vi "Stop_queue.vi"(7 "Refs cluster In":T1) -> ()   [LabVIEW 2015]
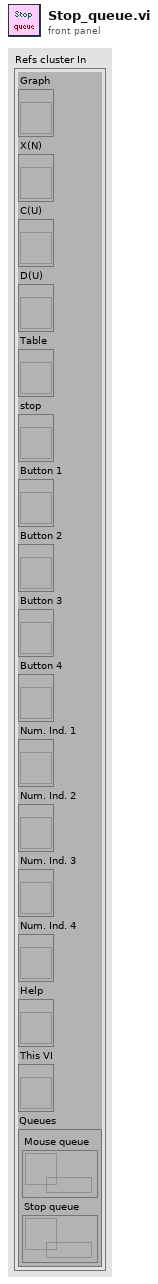
[diagram p1: front panel]
types:
  T1 = cluster{"Graph":refnum<vi>, "X(N)":refnum<vi>, "C(U)":refnum<vi>, "D(U)":refnum<vi>, "Table":refnum<vi>, "stop":refnum<vi>, "Button 1":refnum<vi>, "Button 2":refnum<vi>, "Button 3":refnum<vi>, "Button 4":refnum<vi>, "Num. Ind. 1":refnum<vi>, "Num. Ind. 2":refnum<vi>, "Num. Ind. 3":refnum<vi>, "Num. Ind. 4":refnum<vi>, "Help":refnum<vi>, "This VI":refnum<vi>, "Queues":cluster{"Mouse queue":refnum<queue>, "Stop queue":refnum<queue>}}
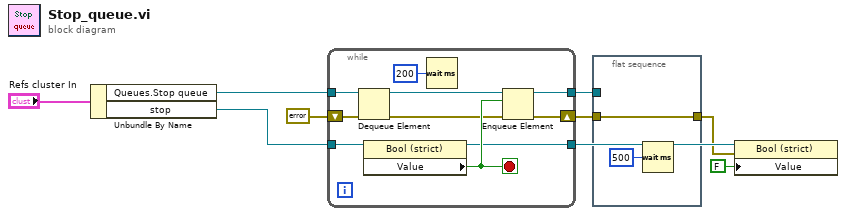
[diagram p0: block diagram]
diagram:
  n1 = Unbundle By Name("Refs cluster In") -> ("Queues.Stop queue"=w2:refnum<queue>, "stop"=w1:refnum<vi>)
  n2 = while {
    tunnel: w2 -> [w19]
    tunnel: [w17] -> w5
    tunnel: w1 -> [w14]
    tunnel: [w12] -> w8
    shift-right: [w16] -> w6
    shift-left: errorcluster {"status"=FALSE, "code"=0, "source"=""} ("error in") -> [w15]
    stop <- w13 stop-if-true
    n3 = Dequeue Element(queue=w19, error in (no error)=w15) -> (queue out=w18:refnum<queue>, error out=w11:errorcluster)  [unwired: 1 in, 2 out]
    n4 = property class="Bool (strict)"(reference=w14) -> (reference out=w12:refnum<vi>, "Value"=w13:bool)  [unwired: 1 in, 1 out]
    n5 = Wait (ms)(milliseconds to wait=u32 200) -> ()  [unwired: 1 out]
    n6 = Enqueue Element(queue=w18, element=w13, error in (no error)=w11) -> (queue out=w17:refnum<queue>, error out=w16:errorcluster)  [unwired: 1 in, 1 out]
  }
  n7 = flat-sequence {
    tunnel: w6 -> [w20]
    tunnel: w5 -> [_]
    tunnel: [w20] -> w4
    frame #0 {
      n8 = Wait (ms)(milliseconds to wait=u32 500) -> ()  [unwired: 1 out]
    }
  }
  n9 = property class="Bool (strict)"(reference=w8, error in=w4, "Value"=FALSE) -> ()  [unwired: 2 out]
